vi "testSlave.vi"() -> ()   [LabVIEW 2015]
uses:
  NetworkStream/NetworkStreamReceiverState.ctl
  NetworkStream/NetworkStreamStateMachineVariable.ctl
  NetworkStream/NetworkStreamData.ctl
  <vilib>/dex/Stream Element Allocation Mode.ctl
  NetworkStream/NetworkStream.lvlib
panel:
  out "data":dbl
  in  "Stop Button 2":bool
  out "Session Hash 2":u64
  out "Network Stream State Indicator 2":T1
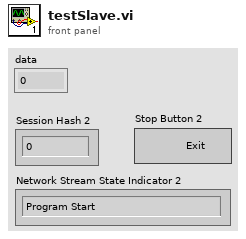
[diagram p1: front panel]
types:
  T1 = typedef "NetworkStream.lvlib/NetworkStreamReceiverState.ctl" = enum16{"Program Start", "Waiting for connection", "Connected", "Connection lost", "Exit", "Unhandled Exception"}
  T2 = typedef "NetworkStream.lvlib/NetworkStreamData.ctl" = cluster{"Command/Status":string, "Data":variant, "Session Hash":u64, "Sequence Number":u64}
  T3 = typedef "NetworkStream.lvlib/NetworkStreamStateMachineVariable.ctl" = cluster{"Network Stream Reader Endpoint":refnum<k21>, "Last Received Sequence Number":u64}
  T4 = typedef "Stream Element Allocation Mode.ctl" = u32
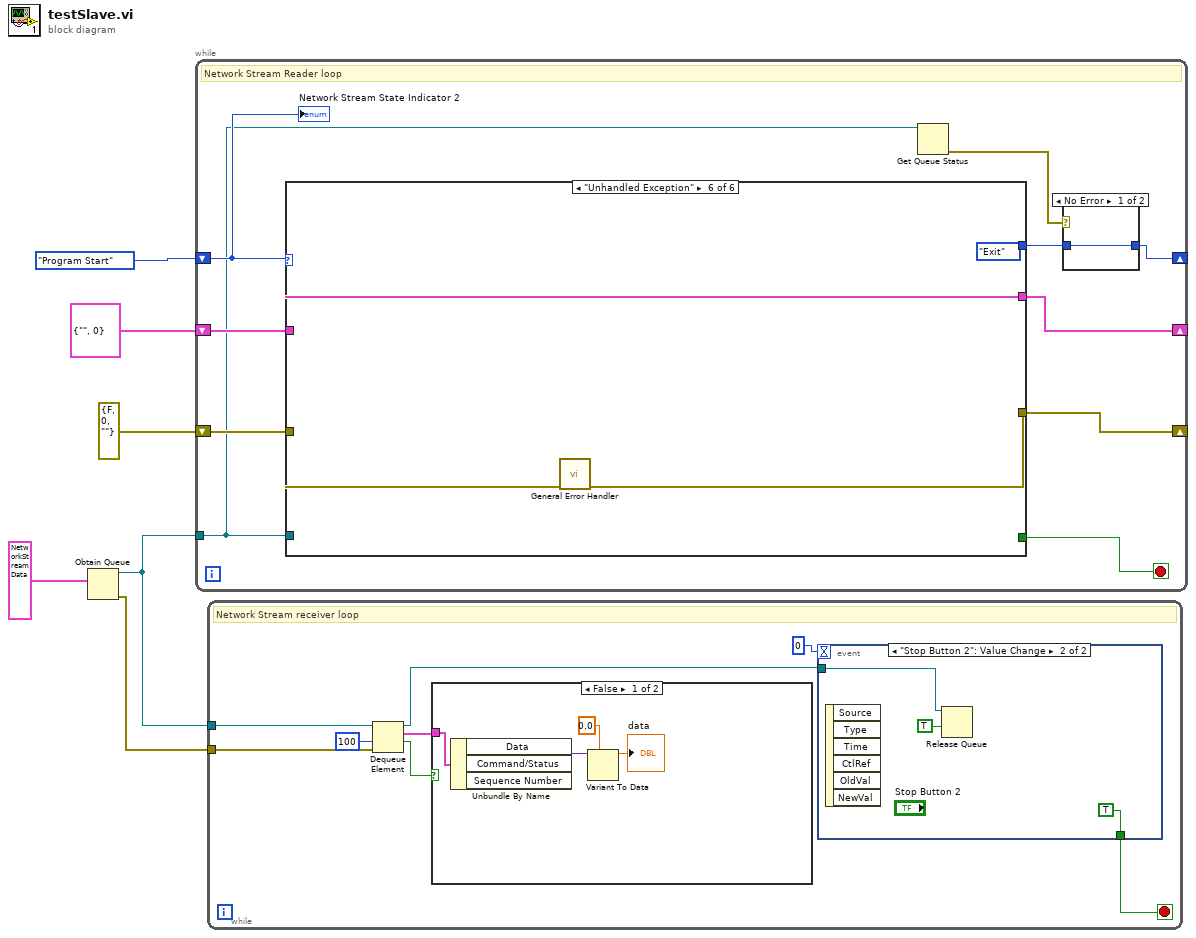
[diagram p0: block diagram]
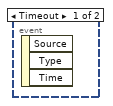
[diagram p3: hidden frame]
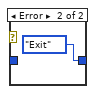
[diagram p4: hidden frame]
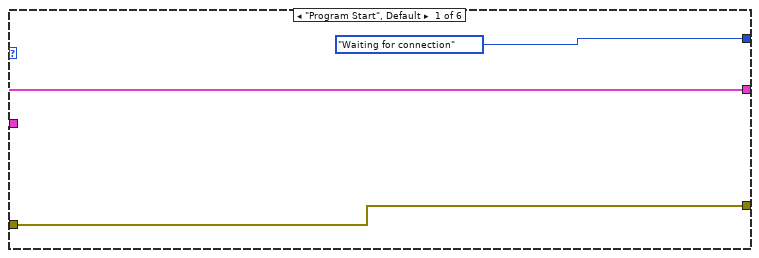
[diagram p5: hidden frame]
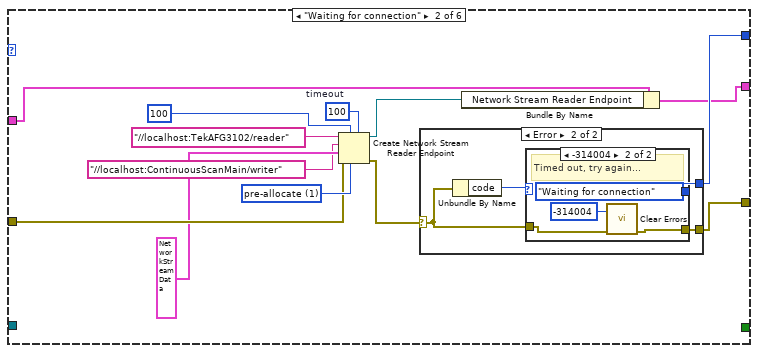
[diagram p6: hidden frame]
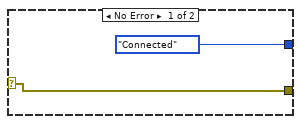
[diagram p7: hidden frame]
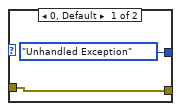
[diagram p8: hidden frame]
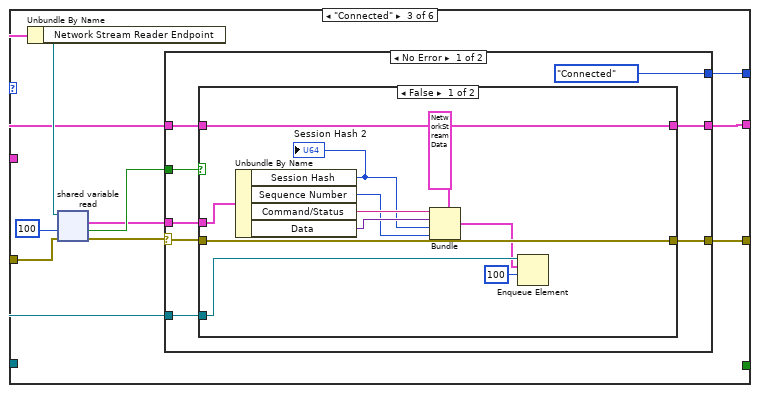
[diagram p9: hidden frame]
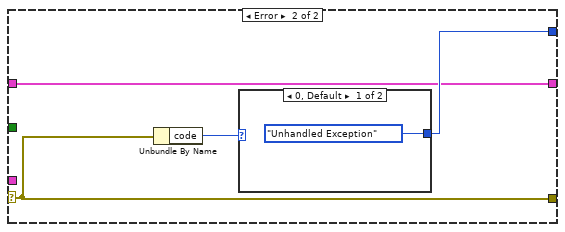
[diagram p11: hidden frame]
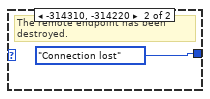
[diagram p12: hidden frame]
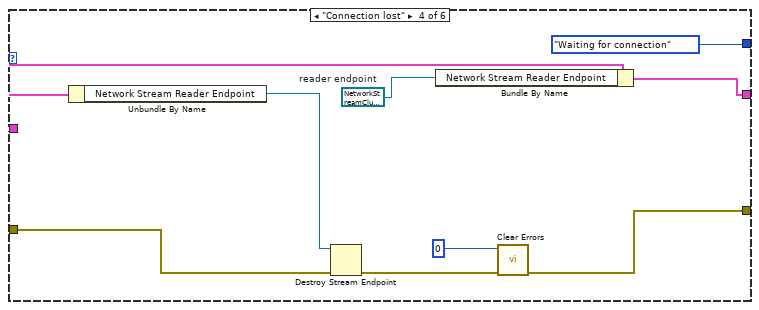
[diagram p13: hidden frame]
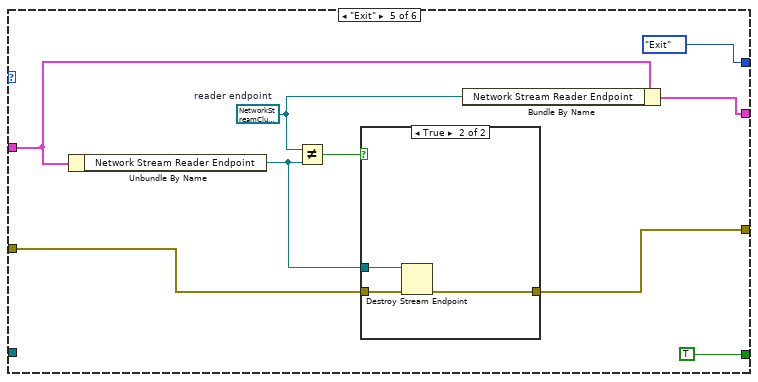
[diagram p14: hidden frame]
diagram:
  n1 = Obtain Queue(element data type=T2 {"Command/Status"="", "Data"=variant, "Session Hash"=0, "Sequence Number"=0} ("NetworkStreamCluster")) -> (queue out=w2:refnum<queue>, error out=w3:errorcluster)  [unwired: 4 in, 1 out]
  n2 = while {
    shift-right: [w14] -> _
    shift-left: T3 {"Network Stream Reader Endpoint"="", "Last Received Sequence Number"=0} ("StateMachineVariable") -> [w16]
    shift-right: [w9] -> _
    shift-left: NetworkStreamReceiverState."Program Start" -> [w15]
    shift-right: [w13] -> _
    shift-left: errorcluster {"status"=FALSE, "code"=0, "source"=""} ("error in (no error)") -> [w11]
    tunnel: w2 -> [w7]
    stop <- w12 stop-if-true
    # "Network Stream Reader loop"
    n3 = case shown="\"Unhandled Exception\"" w15 {
      tunnel: [NetworkStreamReceiverState."Waiting for connection" w30 w52 NetworkStreamReceiverState."Waiting for connection" NetworkStreamReceiverState."Exit" NetworkStreamReceiverState."Exit"] -> w10
      tunnel: [w20 w29 w53 w89 w102 w110] -> w13
      tunnel: [w19 w28 w50 w85 w95 w107] -> w14
      tunnel: [_ _ _ _ TRUE _] -> w12
      tunnel: w16 -> [w19 w26 w49 w86 w96 w107]
      tunnel: w11 -> [w20 w25 w48 w88 w97 w108]
      tunnel: w7 -> [_ _ w47 _ _ _]
      frame "Program Start", Default {
      }
      frame "Waiting for connection" {
        w27 = T4 1 items=["allocate as needed", "pre-allocate"] ("element allocation mode")
        w34 = 100  # timeout
        n4 = Create Network Stream Reader Endpoint(5:w34, 6:w27, 7:100 ("reader buffer size"), 8:w25, 9:T2 {"Command/Status"="", "Data"=variant, "Session Hash"=0, "Sequence Number"=0} ("NetworkStreamCluster"), 10:"//localhost:ContinuousScanMain/writer" ("writer url"), 11:"//localhost:TekAFG3102/reader" ("reader name")) -> (0:w31:errorcluster, 3:w23:refnum<k21>)
        n5 = case shown="Error" w31 {
          selector: w31 -> [w35 w38]
          tunnel: [NetworkStreamReceiverState."Connected" w40] -> w30
          tunnel: [w35 w37] -> w29
          frame No Error {
          }
          frame Error {
            n6 = Unbundle By Name(w38) -> ("code"=w39:i32)
            n7 = case shown="-314004" w39 {
              tunnel: [NetworkStreamReceiverState."Unhandled Exception" NetworkStreamReceiverState."Waiting for connection"] -> w40
              tunnel: w38 -> [w41 w44]
              tunnel: [w41 w43] -> w37
              frame 0, Default {
              }
              frame -314004 {
                # "Timed out, try again..."
                n8 = call <vilib>:"Clear Errors.vi"("error in (no error)"=w44, "specific error code to clear (0: all)"=-314004) -> ("error out"=w43:errorcluster)  [unwired: 4 in, 1 out]
              }
            }
          }
        }
        n9 = Bundle By Name(cluster=w26, "Network Stream Reader Endpoint"=w23) -> (w28:T3)
      }
      frame "Connected" {
        n10 = Unbundle By Name(w49) -> ("Network Stream Reader Endpoint"=w51:refnum<k21>)
        n11 = shared-variable-read(w51, w48, 100 ("timeout ms (-1)")) -> (w54:errorcluster, w56:bool, w55:T2)  [unwired: 1 out]
        n12 = case shown="No Error" w54 {
          selector: w54 -> [w63 w82]
          tunnel: w56 -> [w65 _]
          tunnel: w55 -> [w64 _]
          tunnel: [w62 w82] -> w53
          tunnel: [NetworkStreamReceiverState."Connected" w80] -> w52
          tunnel: [w60 w79] -> w50
          tunnel: w49 -> [w59 w79]
          tunnel: w47 -> [w58 _]
          frame No Error {
            n13 = case shown="False" w65 {
              tunnel: [w72 w78] -> w62
              tunnel: w63 -> [w72 w78]
              tunnel: w64 -> [w76 _]
              tunnel: [w73 w77] -> w60
              tunnel: w59 -> [w73 w77]
              tunnel: w58 -> [w71 _]
              frame False {
                n14 = Unbundle By Name(w76) -> ("Session Hash"=w68:u64, "Sequence Number"=w67:u64, "Command/Status"=w75:string, "Data"=w74:variant)
                "Session Hash 2" <- w68
                n15 = Bundle(cluster=T2 {"Command/Status"="", "Data"=variant, "Session Hash"=0, "Sequence Number"=0} ("NetworkStreamCluster"), "Command/Status"=w75, "Data"=w74, "Session Hash"=w68, "Sequence Number"=w67) -> (w70:T2)
                n16 = Enqueue Element(queue=w71, element=w70, timeout in ms (-1)=100) -> ()  [unwired: 1 in, 3 out]
              }
              frame True {
              }
            }
          }
          frame Error {
            n17 = Unbundle By Name(w82) -> ("code"=w81:i32)
            n18 = case shown="0, Default" w81 {
              tunnel: [NetworkStreamReceiverState."Unhandled Exception" NetworkStreamReceiverState."Connection lost"] -> w80
              frame 0, Default {
              }
              frame -314310, -314220 {
                # "The remote endpoint has been destroyed."
              }
            }
          }
        }
      }
      frame "Connection lost" {
        w92 = refnum<k21> refnum  # reader endpoint
        n19 = Unbundle By Name(w86) -> ("Network Stream Reader Endpoint"=w87:refnum<k21>)
        n20 = Destroy Stream Endpoint(8:w88, 11:w87) -> (0:w91:errorcluster)
        n21 = Bundle By Name(cluster=w86, "Network Stream Reader Endpoint"=w92) -> (w85:T3)
        n22 = call <vilib>:"Clear Errors.vi"("error in (no error)"=w91, "specific error code to clear (0: all)"=0) -> ("error out"=w89:errorcluster)  [unwired: 4 in, 1 out]
      }
      frame "Exit" {
        w98 = refnum<k21> refnum  # reader endpoint
        n23 = Unbundle By Name(w96) -> ("Network Stream Reader Endpoint"=w94:refnum<k21>)
        n24 = Not Equal?(x=w98, y=w94) -> (x != y?=w100:bool)
        n25 = case shown="True" w100 {
          tunnel: [w103 w106] -> w102
          tunnel: w97 -> [w103 w105]
          tunnel: w94 -> [_ w104]
          frame False {
          }
          frame True {
            n26 = Destroy Stream Endpoint(8:w105, 11:w104) -> (0:w106:errorcluster)
          }
        }
        n27 = Bundle By Name(cluster=w96, "Network Stream Reader Endpoint"=w98) -> (w95:T3)
      }
      frame "Unhandled Exception" {
        n28 = call <vilib>:"General Error Handler.vi"("error in (no error)"=w108) -> ("error out"=w110:errorcluster)  [unwired: 10 in, 4 out]
      }
    }
    n29 = Get Queue Status(queue=w7) -> (error out=w8:errorcluster)  [unwired: 2 in, 7 out]
    n30 = case shown="No Error" w8 {
      tunnel: w10 -> [w17 _]
      tunnel: [w17 NetworkStreamReceiverState."Exit"] -> w9
      frame No Error {
      }
      frame Error {
      }
    }
    "Network Stream State Indicator 2" <- w15
  }
  n31 = while {
    tunnel: w3 -> [w112]
    tunnel: w2 -> [w113]
    stop <- w118 stop-if-true
    # "Network Stream receiver loop"
    n32 = Dequeue Element(queue=w113, timeout in ms (-1)=100, error in (no error)=w112) -> (queue out=w114:refnum<queue>, element=w116:T2, timed out?=w111:bool)  [unwired: 1 out]
    n33 = case shown="False" w111 {
      tunnel: w116 -> [w122 _]
      frame False {
        n34 = Unbundle By Name(w122) -> ("Data"=w121:variant)  [unwired: 2 out]
        n35 = Variant To Data(type=0.0, Variant=w121) -> (data=→"data":dbl)  [unwired: 1 in, 1 out]
      }
      frame True {
      }
    }
    n36 = event shown="[1] \"Stop Button 2\": Value Change" {
      selector: _ -> [_ _]
      dyn-events: _ -> [_ _]
      timeout: 0 -> [_ _]
      tunnel: [_ TRUE] -> w118
      tunnel: w114 -> [_ w124]
      event Timeout {
        n37 = event-data() -> ()  [unwired: 1 in, 3 out]
      }
      event "Stop Button 2": Value Change {
        n38 = event-data() -> ()  [unwired: 1 in, 6 out]
        n39 = Release Queue(queue=w124, force destroy? (F)=TRUE) -> ()  [unwired: 1 in, 3 out]
      }
    }
  }
